vi "Main - Event Log (eFGV).vi"(7 "Action":T1, 8 "error in":errorcluster, 10 "Fileid":string, 11 "Data In":string) -> (0 "error out":errorcluster, 1 "body":string, 2 "Event":refnum<user-event>, 3 "Data Out":string)   [LabVIEW 2019]
uses:
  Controls/eFGV States.ctl
  <vilib>/httpClient/ClientHandle.ctl
  <vilib>/httpClient/POSTBuffer.vi
  <vilib>/httpClient/LabVIEWHTTPClient.lvlib
panel:
  out "Fileid Out":string
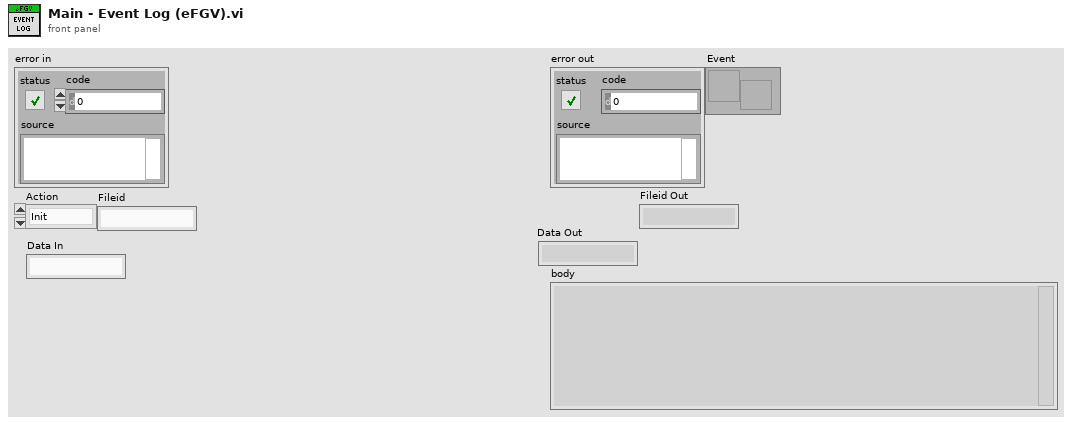
[diagram p1: front panel]
types:
  T1 = typedef "eFGV States.ctl" = enum16{"Init", "Read", "Write", "Exit"}
  T2 = cluster{"action":string, "message":string, "fileid":string}
  T3 = cluster{"status":string, "data":cluster{"created_date":string, "message":string}[]}
  T4 = typedef "LabVIEWHTTPClient.lvlib/ClientHandle.ctl" = refnum<k1>
  T5 = cluster{"created_date":string, "message":string}[]
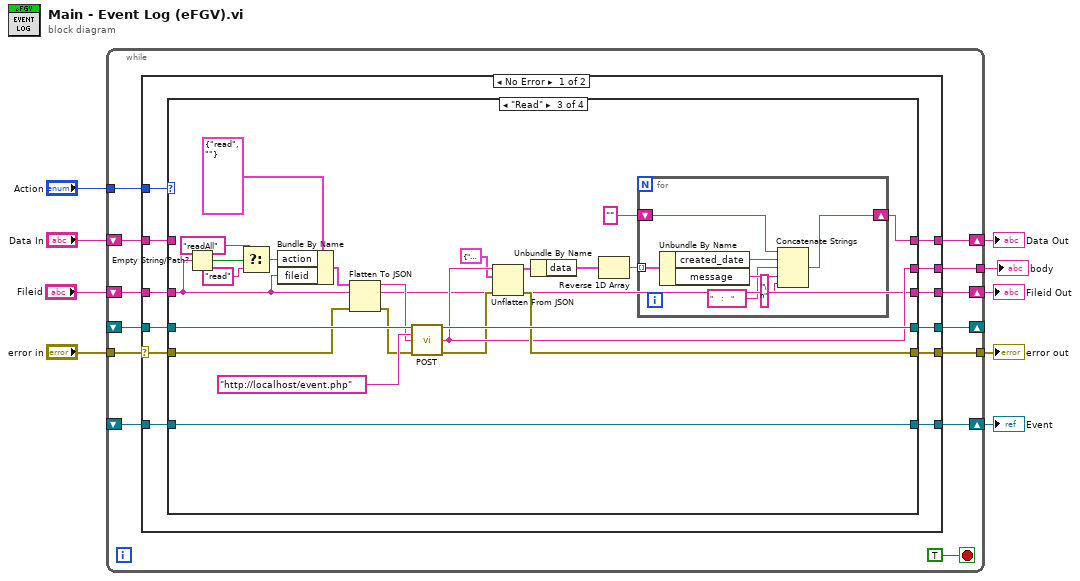
[diagram p0: block diagram]
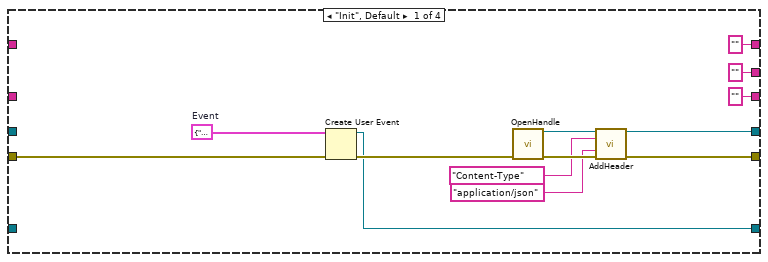
[diagram p2: hidden frame]
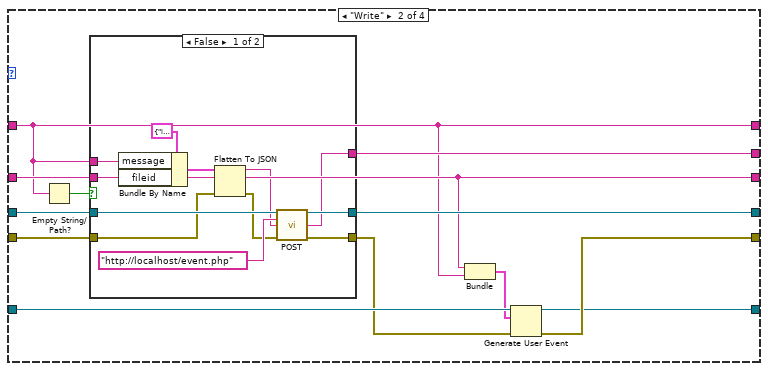
[diagram p3: hidden frame]
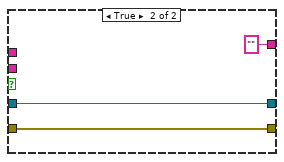
[diagram p4: hidden frame]
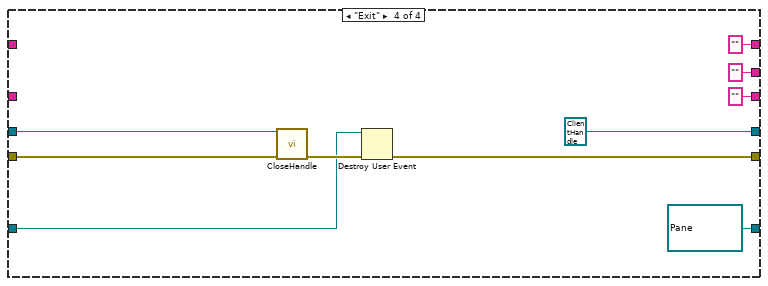
[diagram p5: hidden frame]
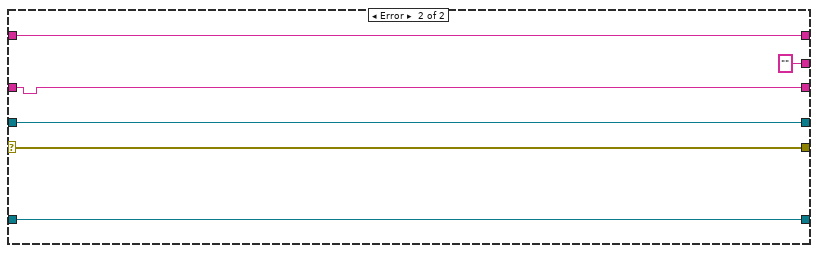
[diagram p6: hidden frame]
diagram:
  n1 = while {
    tunnel: "error in" -> [w21]
    tunnel: [w20] -> w8
    tunnel: "Action" -> [w19]
    shift-right: [w17] -> w5
    shift-left: "Data In" -> [w18]
    shift-right: [w16] -> _
    shift-left: _ -> [w15]
    tunnel: [w14] -> w4
    shift-right: [w12] -> w2
    shift-left: "Fileid" -> [w13]
    shift-right: [w11] -> w1
    shift-left: _ -> [w10]
    stop <- TRUE stop-if-true
    n2 = case shown="No Error" w21 {
      selector: w21 -> [w33 w120]
      tunnel: [w34 w120] -> w20
      tunnel: w19 -> [w32 _]
      tunnel: w18 -> [w31 w119]
      tunnel: [w30 w119] -> w17
      tunnel: [w29 w118] -> w16
      tunnel: w15 -> [w28 w118]
      tunnel: [w27 "" ("body")] -> w14
      tunnel: w10 -> [w26 w116]
      tunnel: w13 -> [w25 w115]
      tunnel: [w24 w115] -> w12
      tunnel: [w23 w116] -> w11
      frame No Error {
        n3 = case shown="\"Read\"" w32 {
          tunnel: [w43 w53 w94 w108] -> w34
          tunnel: w33 -> [w38 w57 w95 w114]
          tunnel: w31 -> [_ w50 _ _]
          tunnel: ["" ("Data In") w50 w93 "" ("Data In")] -> w30
          tunnel: [w42 w58 w96 T4 refnum ("client handle out")] -> w29
          tunnel: w28 -> [_ w59 w97 w113]
          tunnel: ["" ("body") w56 w92 "" ("body")] -> w27
          tunnel: w26 -> [_ w55 w91 w107]
          tunnel: w25 -> [_ w51 w75 _]
          tunnel: ["" ("Fileid") w51 w75 "" ("Fileid")] -> w24
          tunnel: [w35 w48 w91 refnum<user-event> refnum ("Event")] -> w23
          frame "Init", Default {
            w36 = cluster{"fileid":string, "message":string} {"fileid"="", "message"=""}  # Event
            n4 = Create User Event(user event datatype=w36, error in=w38) -> (user event=w35:refnum<user-event>, error out=w39:errorcluster)
            n5 = call <vilib>:"OpenHandle.vi"("error in (no error)"=w39) -> ("client handle out"=w46:T4, "error out"=w47:errorcluster)  [unwired: 13 in]
            n6 = call <vilib>:"AddHeader.vi"("client handle"=w46, "header"="Content-Type", "value"="application/json", "error in (no error)"=w47) -> ("client handle out"=w42:T4, "error out"=w43:errorcluster)  [unwired: 10 in]
          }
          frame "Write" {
            n7 = Empty String/Path?(string/path=w50) -> (empty?=w52:bool)
            n8 = case shown="False" w52 {
              tunnel: w59 -> [w71 w73]
              tunnel: [w70 w73] -> w58
              tunnel: w57 -> [w67 w72]
              tunnel: [w63 "" ("body")] -> w56
              tunnel: [w62 w72] -> w54
              tunnel: w50 -> [w61 _]
              tunnel: w51 -> [w60 _]
              frame False {
                n9 = Bundle By Name(cluster=T2 {"action"="insert", "message"="", "fileid"=""}, "message"=w61, "fileid"=w60) -> (w64:T2)
                n10 = Flatten To JSON(anything=w64, error in (no error)=w67) -> (JSON string=w66:string, 11:w68:errorcluster)  [unwired: 1 in]
                n11 = call-poly <vilib>:"POST.vi"("client handle"=w71, "url"="http://localhost/event.php", "buffer"=w66, "error in (no error)"=w68) -> ("client handle out"=w70:T4, "body"=w63:string, "error out"=w62:errorcluster)  [unwired: 8 in, 1 out]
              }
              frame True {
              }
            }
            n12 = Bundle("Fileid"=w51, "Data In"=w50) -> (w49:cluster{"Fileid":string, "Data In":string})  [unwired: 1 in]
            n13 = Generate User Event(user event=w55, event data cluster=w49, error in=w54) -> (user event out=w48:refnum<user-event>, error out=w53:errorcluster)  [unwired: 1 in]
          }
          frame "Read" {
            n14 = Empty String/Path?(string/path=w75) -> (empty?=w79:bool)
            n15 = Select(t="readAll", s=w79, f="read" ("action")) -> (s? t:f=w76:string)
            n16 = Bundle By Name(cluster=cluster{"action":string, "fileid":string} {"action"="read", "fileid"=""}, "action"=w76, "fileid"=w75) -> (w80:cluster{"action":string, "fileid":string})
            n17 = Flatten To JSON(anything=w80, error in (no error)=w95) -> (JSON string=w88:string, 11:w89:errorcluster)  [unwired: 1 in]
            n18 = call-poly <vilib>:"POST.vi"("client handle"=w97, "url"="http://localhost/event.php", "buffer"=w88, "error in (no error)"=w89) -> ("client handle out"=w96:T4, "body"=w92:string, "error out"=w87:errorcluster)  [unwired: 8 in, 1 out]
            n19 = Unflatten From JSON(JSON string=w92, type and defaults=T3 {"status"="read", "data"=[]}, error in (no error)=w87) -> (value=w85:T3, error out=w94:errorcluster)  [unwired: 4 in]
            n20 = Unbundle By Name(w85) -> ("data"=w84:T5)
            n21 = Reverse 1D Array(array=w84) -> (reversed array=w82:T5)
            n22 = for {
              tunnel: w82 -> [w104] mode=indexing
              shift-right: [w98] -> w93
              shift-left: "" -> [w100]
              n23 = Unbundle By Name(w104) -> ("created_date"=w103:string, "message"=w102:string)
              n24 = Concatenate Strings(w100, w103, "    :    " ("string"), w102, "\n" ("string")) -> (w98:string)
            }
          }
          frame "Exit" {
            n25 = call <vilib>:"CloseHandle.vi"("client handle"=w113, "error in (no error)"=w114) -> ("error out"=w109:errorcluster)  [unwired: 13 in]
            n26 = Destroy User Event(user event=w107, error in=w109) -> (error out=w108:errorcluster)
          }
        }
      }
      frame Error {
      }
    }
  }
  "error out" <- w8
  "Data Out" <- w5
  "body" <- w4
  "Fileid Out" <- w2
  "Event" <- w1
